vi "command.vi"(2 "Direction":string, 7 "LabVIEW Web Service Request":refnum<class "Web Request.lvclass">) -> ()   [LabVIEW 2014]
uses:
  <vilib>/wsapi/Web Request.lvclass
  controls/UI DataSam.ctl
panel:
  # "Use the Web Service Request input terminal to call the VIs on the Web Services palette. Do not remove it from the connector pane unless you don't need access to the palette."
  # "Each additional control wired to the connector pane will be available as an input in the URL. To include an indicator in terminal-mode output (the default setting), it must also be wired to the connector pane."
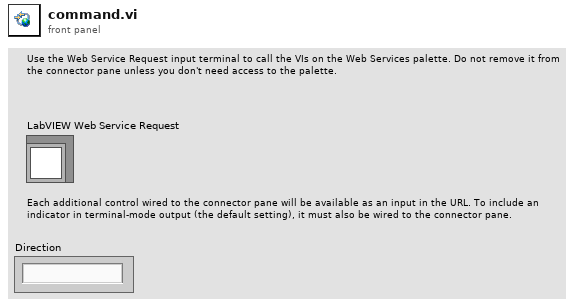
[diagram p1: front panel]
types:
  T1 = typedef "UI DataSam.ctl" = cluster{"Message":string, "Data":variant}
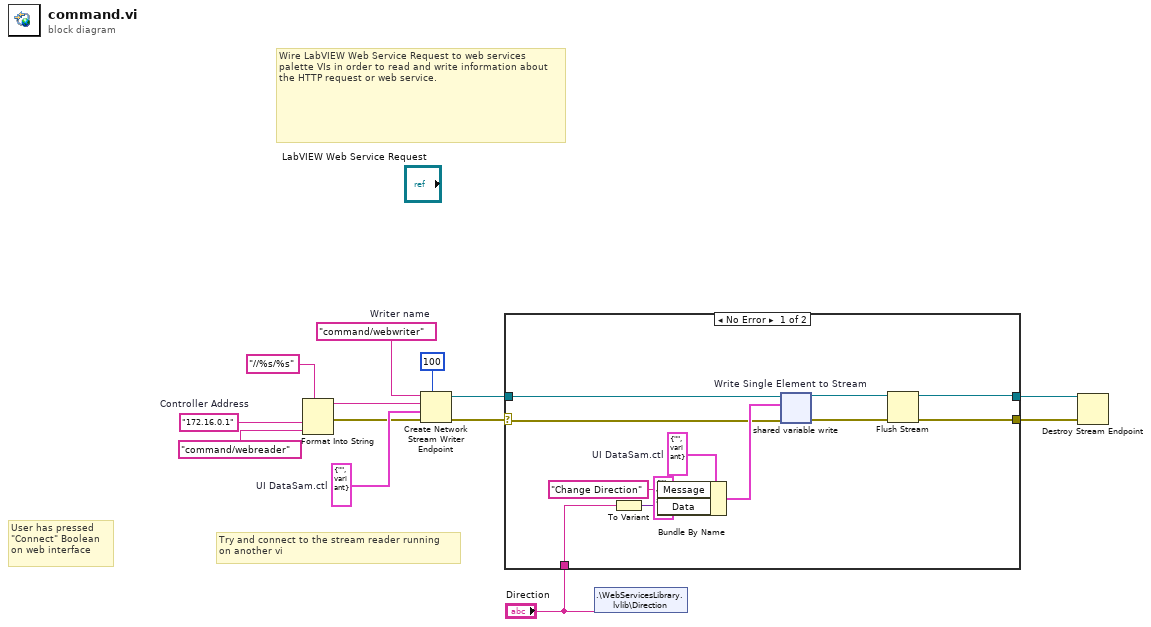
[diagram p0: block diagram]
diagram:
  w13 = "172.16.0.1"  # Controller Address
  w10 = T1 {"Message"="", "Data"=variant}  # UI DataSam.ctl
  w9 = "command/webwriter"  # Writer name
  (unwired) T1 {"Message"="", "Data"=variant} ("UI DataSam.ctl")
  # "Try and connect to the stream reader running\non another vi"
  # "User has pressed\n\"Connect\" Boolean\non web interface"
  # "Wire LabVIEW Web Service Request to web services palette VIs in order to read and write information about the HTTP request or web service."
  n1 = Format Into String(format string="//%s/%s", w13, "command/webreader" ("input 2")) -> (resulting string=w7:string, error out=w6:errorcluster)  [unwired: 2 in]
  n2 = Create Network Stream Writer Endpoint(7:100 ("writer buffer size"), 8:w6, 9:w10, 10:w7, 11:w9) -> (0:w12:errorcluster, 3:w11:refnum<k21>)  [unwired: 2 in]
  n3 = case shown="No Error" w12 {
    selector: w12 -> [w15 w25]
    tunnel: w11 -> [w20 w26]
    tunnel: [w19 w26] -> w3
    tunnel: [w18 w25] -> w2
    tunnel: "Direction" -> [w14 _]
    frame No Error {
      w17 = T1 {"Message"="", "Data"=variant}  # UI DataSam.ctl
      n4 = To Variant(anything=w14) -> (Variant=w24:variant)
      n5 = Bundle By Name(cluster=w17, "Message"="Change Direction", "Data"=w24) -> (w16:T1)
      n6 = shared-variable-write "Write Single Element to Stream"(w20, w15, w16) -> (w22:refnum<k21>, w21:errorcluster)  [unwired: 1 in, 1 out]
      n7 = Flush Stream(8:w21, 11:w22) -> (0:w18:errorcluster, 3:w19:refnum<k21>)  [unwired: 2 in, 1 out]
    }
    frame Error {
    }
  }
  n8 = shared-variable ".\\WebServicesLibrary.lvlib\\Direction"("Direction") -> ()  [unwired: 1 in, 1 out]
  n9 = Destroy Stream Endpoint(8:w2, 11:w3) -> ()  [unwired: 1 out]
